vi "View Front Panel.vi"(8 "error in (no error)":errorcluster, 10 "SubPnl Refnum":refnum<vi>, 11 "MFC in":refnum<class "MFC.lvclass">) -> (0 "error out":errorcluster, 3 "MFC out":refnum<class "MFC.lvclass">)   [LabVIEW 2013]
uses:
  MFC.lvclass
  PluginInterface/PluginInterface.lvlibp/PluginInterfaceClass/Read VI Refnum.vi
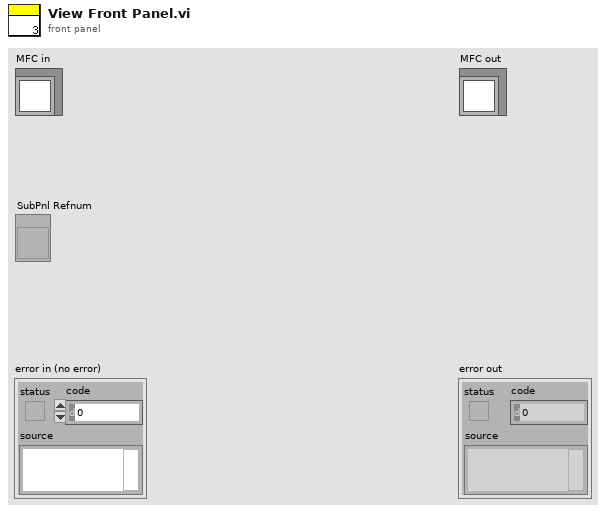
[diagram p1: front panel]
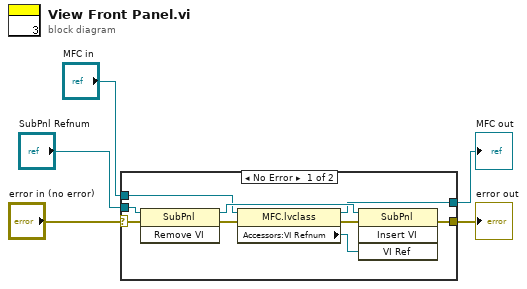
[diagram p0: block diagram]
diagram:
  n1 = case shown="No Error" "error in (no error)" {
    selector: "error in (no error)" -> [w12 w16]
    tunnel: [w14 w16] -> w3
    tunnel: [w9 w15] -> w2
    tunnel: "MFC in" -> [w10 w15]
    tunnel: "SubPnl Refnum" -> [w13 _]
    frame No Error {
      n2 = invoke class="SubPnl" method="Remove VI"(reference=w13, error in=w12) -> (reference out=w11:refnum<vi>, error out=w8:errorcluster)  [unwired: 1 in, 1 out]
      n3 = property class="MFC.lvclass"(reference=w10, error in=w8) -> (reference out=w9:refnum<class "MFC.lvclass">, error out=w7:errorcluster, "Accessors:VI Refnum"=w6:refnum<vi>)
      n4 = invoke class="SubPnl" method="Insert VI"(reference=w11, error in=w7, "VI Ref"=w6) -> (error out=w14:errorcluster)  [unwired: 1 in, 3 out]
    }
    frame Error {
    }
  }
  "error out" <- w3
  "MFC out" <- w2
